vi "Read Fault List.vi"(8 "error in":errorcluster, 9 "timeout (-1)":i32=-1, 11 "Standard Engine Runtime in":refnum<class "Standard Engine Runtime.lvclass">) -> (0 "error out":errorcluster, 2 "faults":T1[](array[typedef]), 3 "Standard Engine Runtime out":refnum<class "Standard Engine Runtime.lvclass">)   [LabVIEW 2013, in "Standard Engine Runtime.lvclass"]
doc: "Retrieves all uncleared faults from the engine. Faults are any recoverable errors which did not result in engine shutdown."
uses:
  Standard Engine Runtime.lvclass
  <vilib>/NI/Module Execution Interface/Engine Runtime/Fault.ctl
  <vilib>/NI/Tag Bus Module Framework/runtime/error classification.ctl
  rt fault.ctl
  <vilib>/NI/Tag Bus Module Framework/module configuration/TBM module configuration.lvclass
  Standard Engine Runtime.lvclass/Standard Engine Runtime.ctl
  <vilib>/NI/Tag Bus Module Framework/runtime/TBM module execution interface.lvclass
  main engine/main engine.lvlib
  <vilib>/NI/Module Execution Interface/Engine Runtime/Engine Runtime Interface.lvclass
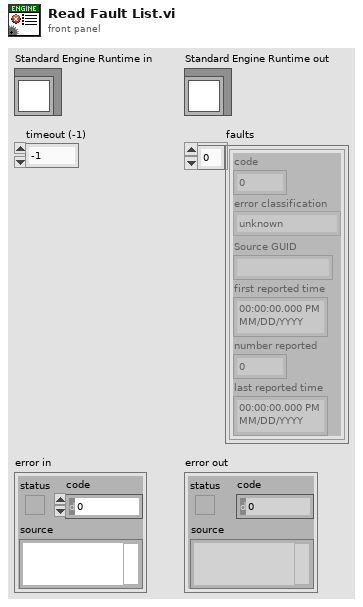
[diagram p1: front panel]
types:
  T1 = typedef "Engine Runtime Interface.lvclass/Fault.ctl" = cluster{"code":i32, "error classification":T2, "Source GUID":string, "first reported time":timestamp, "number reported":u32, "last reported time":timestamp}
  T2 = typedef "TBM module execution interface.lvclass/error classification.ctl" = enum16{"unknown", "none", "trivial", "recoverable", "critical"}
  T3 = typedef "main engine.lvlib/rt fault.ctl" = cluster{"code":i32, "classification":T2, "iteration":u64, "cfg ref":refnum<data-value>}
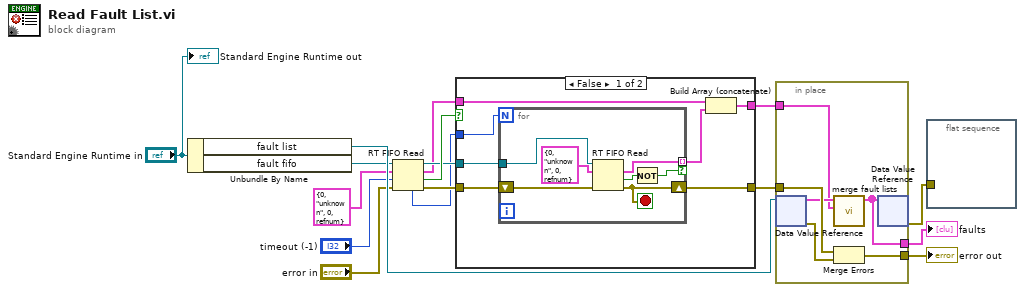
[diagram p0: block diagram]
diagram:
  n1 = Unbundle By Name("Standard Engine Runtime in") -> ("fault list"=w15:refnum<data-value>, "fault fifo"=w11:refnum<k33>)
  n2 = RT FIFO Read(0:w11, 1:T3 {"code"=0, "classification"=enum."unknown", "iteration"=0, "cfg ref"=refnum} ("element"), 2:"timeout (-1)", 3:"error in") -> (7:w1:u32, 8:w3:refnum<k33>, 9:w2:T3, 10:w7:bool, 11:w6:errorcluster)
  n3 = case shown="False" w7 {
    tunnel: w6 -> [w20 w31]
    tunnel: [w19 w31] -> w5
    tunnel: [w17 _] -> w4
    tunnel: w3 -> [w21 _]
    tunnel: w2 -> [w22 _]
    tunnel: w1 -> [w23 _]
    frame False {
      n4 = for {
        N: w23 -> [_]
        tunnel: w21 -> [w30]
        tunnel: [w28] -> w18 mode=indexing if=w25
        shift-right: [w24] -> w19
        shift-left: w20 -> [w27]
        stop <- w24 stop-if-true
        n5 = RT FIFO Read(0:w30, 1:T3 {"code"=0, "classification"=enum."unknown", "iteration"=0, "cfg ref"=refnum} ("element"), 3:w27) -> (9:w28:T3, 10:w26:bool, 11:w24:errorcluster)  [unwired: 1 in, 2 out]
        n6 = Not(x=w26) -> (.not. x?=w25:bool)
      }
      n7 = Build Array (concatenate)(w22, w18) -> (w17:T3[])
    }
    frame True {
    }
  }
  n8 = in-place {
    in-place-border: w5 -> [w37]
    in-place-border: [w35] -> w13
    in-place-border: [w33] -> w12
    in-place-border: w4 -> [w32]
    n9 = in-place-dvr #1(w15) -> (w34:T1[], w36:errorcluster)
    n10 = call "merge fault lists.vi"("rt faults"=w32, "faults in"=w34) -> ("faults out"=w33:T1[])  [unwired: 9 in]
    n11 = Merge Errors(w37, w36) -> (w35:errorcluster)
    n12 = in-place-dvr #1(w33) -> (w14:errorcluster)  [unwired: 1 out]
  }
  "error out" <- w13
  "faults" <- w12
  n13 = flat-sequence {
    tunnel: w14 -> [_]
    frame #0 {
    }
  }
  "Standard Engine Runtime out" <- "Standard Engine Runtime in"
